vi "Energize.vi"(8 "error in (no error)":errorcluster, 11 "CIFPlugin in":refnum<class "Template_Plugin.lvclass">) -> (0 "error out":errorcluster, 3 "CIFPlugin out":refnum<class "Template_Plugin.lvclass">)   [LabVIEW 2021, in "Template_Plugin.lvlib"]
uses:
  Template_Plugin.lvlib
  <vilib>/CIF Foundation/CIF Core/CIFCore/Class/CIFCorePlugin.lvclass
  Class/Template_Plugin.lvclass
  C:/Program Files/National Instruments/LabVIEW 2021/vi.lib/CIF Foundation/CIF Core/CIFCore/Class/CIFCorePlugin.lvclass
  D:/dev/Plugins/Template/src/Source/CIF/Plugin Generator/Template/Class/Template_Plugin.lvclass
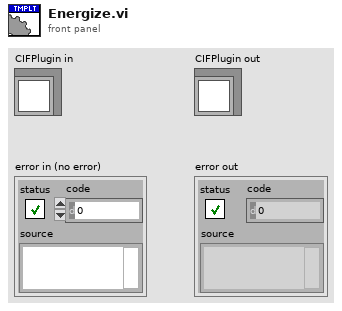
[diagram p1: front panel]
types:
  T1 = typedef "CIFCorePlugin.lvclass/Prepare State Logic.ctl" = enum16{"Listen", "Prepare", "Error", "Destroy"}
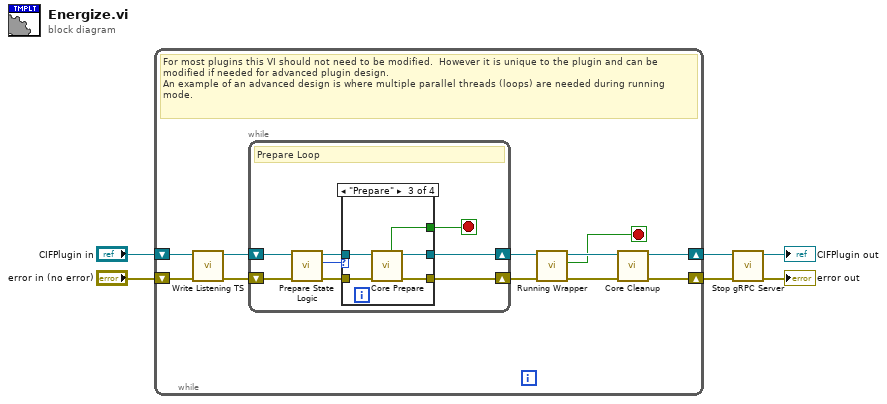
[diagram p0: block diagram]
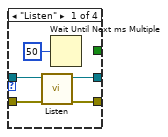
[diagram p2: hidden frame]
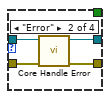
[diagram p3: hidden frame]
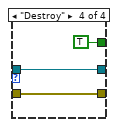
[diagram p4: hidden frame]
diagram:
  n1 = while {
    shift-right: [w17] -> w5
    shift-left: "CIFPlugin in" -> [w12]
    shift-right: [w16] -> w6
    shift-left: "error in (no error)" -> [w15]
    stop <- w7 stop-if-true
    # "For most plugins this VI should not need to be modified.  However it is unique to the plugin and can be modified if needed for advanced plugin design.  \nAn example of an advanced design is where multiple parallel threads (loops) are needed during running mode."
    n2 = call <vilib>:"Write Listening TS.vi"("error in (no error)"=w15, "CIFCorePlugin in"=w12) -> ("error out"=w13:errorcluster, "CIFCorePlugin out"=w14:refnum<class "Template_Plugin.lvclass">)  [unwired: 8 in]
    n3 = while {
      shift-right: [w25] -> w10
      shift-left: w14 -> [w18]
      shift-right: [w20] -> w11
      shift-left: w13 -> [w21]
      stop <- w19 stop-if-true
      # "Prepare Loop"
      n4 = call <vilib>:"Prepare State Logic.vi"("error in (no error)"=w21, "CIFCorePlugin in"=w18) -> ("error out"=w22:errorcluster, "Prepare State Logic"=w23:T1, "CIFCorePlugin out"=w24:refnum<class "Template_Plugin.lvclass">)  [unwired: 7 in]
      n5 = case shown="\"Prepare\"" w23 {
        tunnel: [w26 w34 w39 w42] -> w25
        tunnel: w24 -> [w28 w31 w35 w42]
        tunnel: w22 -> [w29 w32 w36 w41]
        tunnel: [w27 w33 w38 w41] -> w20
        tunnel: [_ _ w37 TRUE ("Transition to Run")] -> w19
        frame "Listen" {
          n6 = call-dynamic "Listen.vi"("error in (no error)"=w29, "CIFPlugin in"=w28) -> ("error out"=w27:errorcluster, "CIFPlugin out"=w26:refnum<class "Template_Plugin.lvclass">)  [unwired: 8 in]
          n7 = Wait Until Next ms Multiple(millisecond multiple=u32 50) -> ()  [unwired: 1 out]
        }
        frame "Error" {
          n8 = call <vilib>:"Core Handle Error.vi"("error in (no error)"=w32, "CIFTemplateNode in"=w31) -> ("error out"=w33:errorcluster, "CIFTemplateNode out"=w34:refnum<class "Template_Plugin.lvclass">)  [unwired: 8 in]
        }
        frame "Prepare" {
          n9 = call <vilib>:"Core Prepare.vi"("error in (no error)"=w36, "CIFTemplateNode in"=w35) -> ("error out"=w38:errorcluster, "CIFTemplateNode out"=w39:refnum<class "Template_Plugin.lvclass">, "Transition to Run"=w37:bool)  [unwired: 7 in]
        }
        frame "Destroy" {
        }
      }
    }
    n10 = call-dynamic "Running Wrapper.vi"("error in (no error)"=w11, "CIFPlugin in"=w10) -> ("error out"=w8:errorcluster, "Destroy"=w7:bool, "CIFPlugin out"=w9:refnum<class "Template_Plugin.lvclass">)  [unwired: 7 in]
    n11 = call <vilib>:"Core Cleanup.vi"("error in (no error)"=w8, "CIFTemplateNode in"=w9) -> ("error out"=w16:errorcluster, "CIFTemplateNode out"=w17:refnum<class "Template_Plugin.lvclass">)  [unwired: 8 in]
  }
  n12 = call <vilib>:"Stop gRPC Server.vi"("error in (no error)"=w6, "CIFCorePlugin in"=w5) -> ("error out"=→"error out":errorcluster, "CIFCorePlugin out"=→"CIFPlugin out":refnum<class "Template_Plugin.lvclass">)  [unwired: 8 in]
